vi "Configure Level.vi"(0 "VISA resource name":refnum<visa-resource-name>, 1 "Reference Level (0)":dbl, 2 "Reference Level Offset (0 dB)":dbl, 5 "Amplitude Units (0: dBm)":u16(ring) items=["dBm", "dBmV", "dBmA", "dBuV", "dBuVm", "dBuA", "dBuAm", "dBpt", "dBg", "Volts", "Watts", "Amps"], 7 "Input Impedance (0: 50 ohms)":u16(ring) items=["50", "75"], 11 "error in (no error)":errorcluster, 12 "Enable Auto Attenuation (T: Enable)":bool=TRUE, 13 "Manual Attenuation (30 dB)":dbl=30.0, 14 "Attenuation Step (2 dB)":i32=2) -> (4 "VISA resource name out":refnum<visa-resource-name>, 15 "error out":errorcluster)   [LabVIEW 2014, in "Agilent ESA PSA Series.lvlib"]
doc: "Configures the vertical settings of the spectrum analyzer."
uses:
  Agilent ESA PSA Series.lvlib
panel:
  # "For PSA"
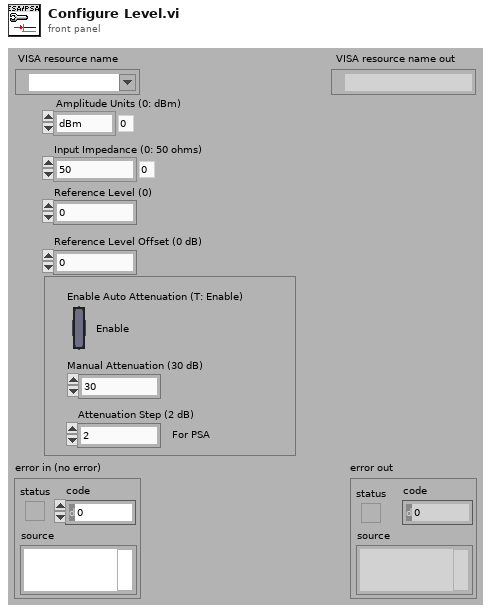
[diagram p1: front panel]
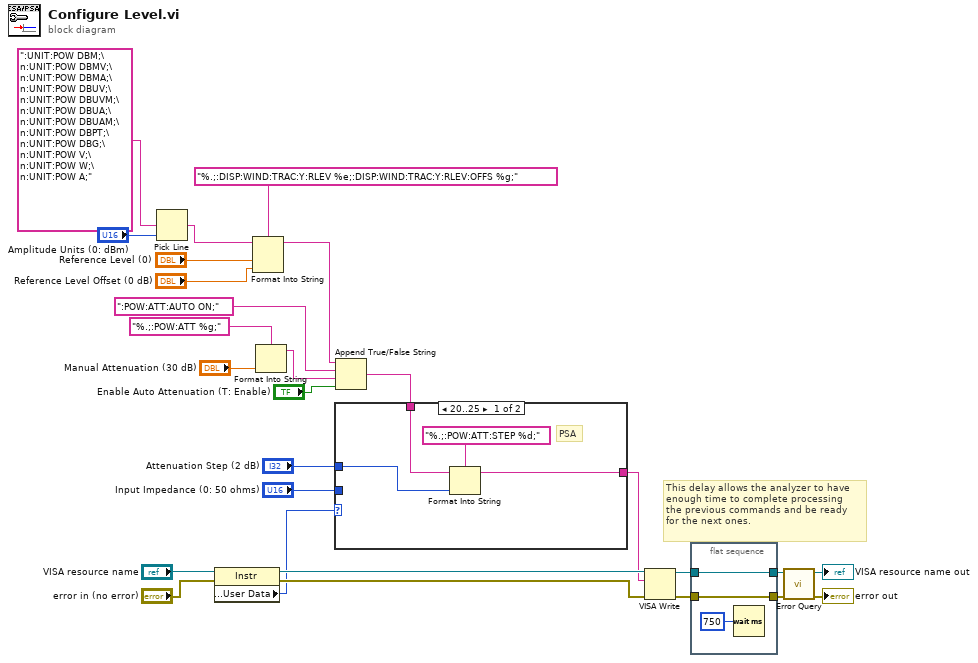
[diagram p0: block diagram]
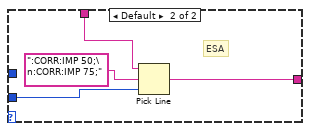
[diagram p2: hidden frame]
diagram:
  # "This delay allows the analyzer to have\nenough time to complete processing\nthe previous commands and be ready\nfor the next ones."
  n1 = Pick Line(multi-line string=":UNIT:POW DBM;\n:UNIT:POW DBMV;\n:UNIT:POW DBMA;\n:UNIT:POW DBUV;\n:UNIT:POW DBUVM;\n:UNIT:POW DBUA;\n:UNIT:POW DBUAM;\n:UNIT:POW DBPT;\n:UNIT:POW DBG;\n:UNIT:POW V;\n:UNIT:POW W;\n:UNIT:POW A;", line index="Amplitude Units (0: dBm)") -> (output string=w16:string)  [unwired: 1 in]
  n2 = property on="Property Node" class="Instr"(reference="VISA resource name", error in="error in (no error)") -> (reference out=w22:refnum<visa-resource-name>, error out=w23:errorcluster, "General Settings:User Data"=w6:u32)
  n3 = Format Into String(format string="%.;:DISP:WIND:TRAC:Y:RLEV %e;:DISP:WIND:TRAC:Y:RLEV:OFFS %g;", initial string=w16, "Reference Level (0)", "Reference Level Offset (0 dB)") -> (resulting string=w9:string)  [unwired: 1 in, 1 out]
  n4 = Format Into String(format string="%.;:POW:ATT %g;", "Manual Attenuation (30 dB)") -> (resulting string=w11:string)  [unwired: 2 in, 1 out]
  n5 = Append True/False String(1:"Enable Auto Attenuation (T: Enable)", 2:w11, 3:":POW:ATT:AUTO ON;" ("string (\"\")"), 4:w9) -> (0:w5:string)
  n6 = case shown="20..25" w6 {
    tunnel: "Input Impedance (0: 50 ohms)" -> [_ w35]
    tunnel: "Attenuation Step (2 dB)" -> [w30 _]
    tunnel: w5 -> [w29 w33]
    tunnel: [w28 w32] -> w7
    frame 20..25 {
      # "PSA"
      n7 = Format Into String(format string="%.;:POW:ATT:STEP %d;", initial string=w29, w30) -> (resulting string=w28:string)  [unwired: 1 in, 1 out]
    }
    frame Default {
      # "ESA"
      n8 = Pick Line(string ("")=w33, multi-line string=":CORR:IMP 50;\n:CORR:IMP 75;", line index=w35) -> (output string=w32:string)
    }
  }
  n9 = VISA Write(VISA resource name=w22, write buffer=w7, error in (no error)=w23) -> (VISA resource name out=w4:refnum<visa-resource-name>, error out=w3:errorcluster)  [unwired: 1 out]
  n10 = flat-sequence {
    tunnel: [w38] -> w2
    tunnel: w4 -> [w38]
    tunnel: [w37] -> w1
    tunnel: w3 -> [w37]
    frame #0 {
      n11 = Wait (ms)(milliseconds to wait=u32 750) -> ()  [unwired: 1 out]
    }
  }
  n12 = call "Error Query.vi"("error in (no error)"=w1, "VISA resource name"=w2) -> ("error out"=→"error out":errorcluster, "VISA resource name out"=→"VISA resource name out":refnum<visa-resource-name>)  [unwired: 6 in, 2 out]
